vi "LJM_AddressesToMBFB.vi"(1 "NumFrames In (Auto-Detect)":i32=-1, 2 "MaxBytesPerPacket":i32, 5 "aAddresses":i32[](array[numeric]), 7 "aTypes":i32[](array[numeric]), 9 "aValuesIn":dbl[](array[numeric]) format="%.2f", 11 "error in":errorcluster, 12 "aWrites":i32[](array[ring]) items=["Read", "Write"], 13 "aNumValues":i32[](array[numeric])) -> (3 "NumFrames Out":i32, 10 "MBFBCommand":u8[](array[numeric]), 15 "error out":errorcluster)   [LabVIEW 2020]
uses:
  LabJackM.framework
panel:
  # "1/20/2015:  Default value of NumFrames changed to -1 which\nequates to Auto-Detect.  If NumFrames = -1, then the NumFrames\ncontrol is ignored and the size of aNames/aAddresses is used to\ndetermine how many frames there are."
  # "0 => 62"
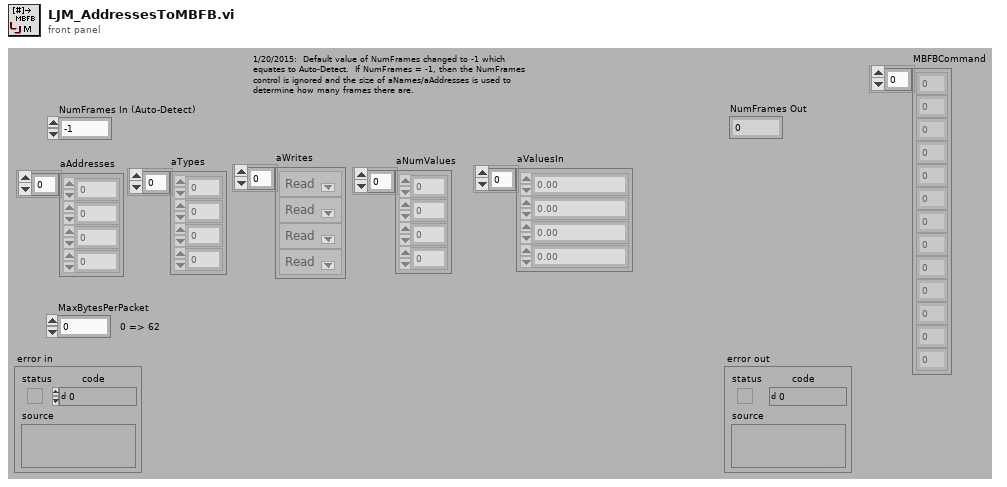
[diagram p1: front panel]
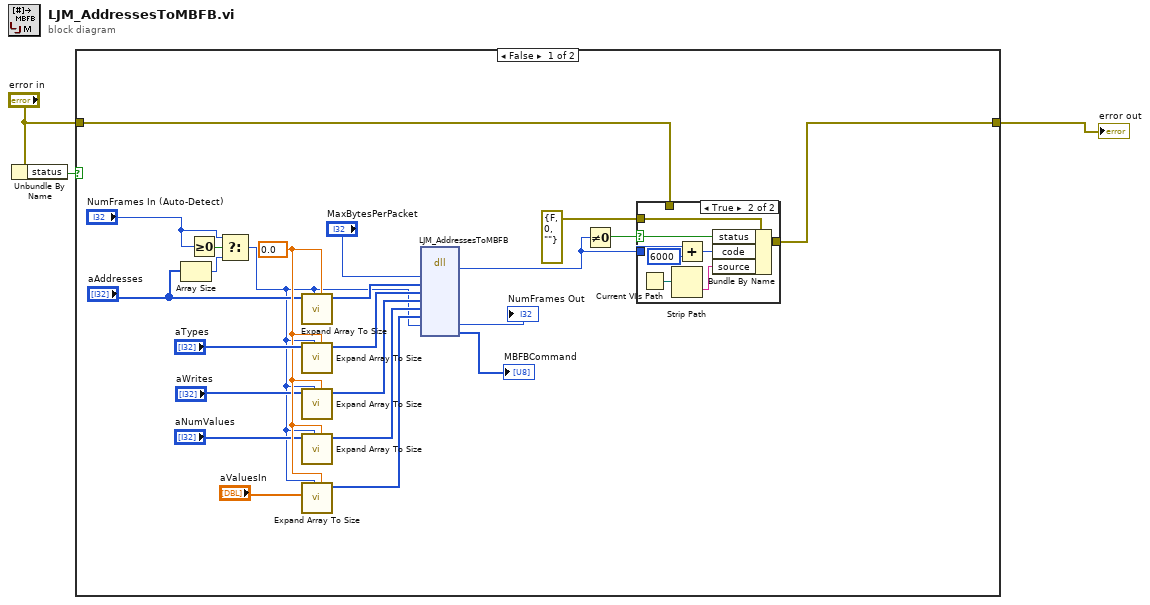
[diagram p0: block diagram]
diagram:
  n1 = Unbundle By Name("error in") -> ("status"=w3:bool)
  n2 = case shown="False" w3 {
    tunnel: "error in" -> [w23 w36]
    tunnel: [w22 w36] -> w1
    frame False {
      w19 = 0.0 ("Default Value")
      n3 = Array Size(array="aAddresses") -> (size(s)=w8:i32)
      n4 = Greater Or Equal To 0?(x="NumFrames In (Auto-Detect)") -> (x >= 0?=w7:bool)
      n5 = Select(t="NumFrames In (Auto-Detect)", s=w7, f=w8) -> (s? t:f=w4:i32)
      n6 = call "Expand Array To Size.vi"("Default Value"=w19, "# Elements"=w4, "I32 Array In"="aAddresses") -> ("I32 Array Out"=w16:i32[])  [unwired: 4 in, 4 out]
      n7 = call "Expand Array To Size.vi"("Default Value"=w19, "# Elements"=w4, "I32 Array In"="aTypes") -> ("I32 Array Out"=w15:i32[])  [unwired: 4 in, 4 out]
      n8 = call "Expand Array To Size.vi"("Default Value"=w19, "# Elements"=w4, "I32 Array In"="aWrites") -> ("I32 Array Out"=w14:i32[])  [unwired: 4 in, 4 out]
      n9 = call "Expand Array To Size.vi"("Default Value"=w19, "# Elements"=w4, "I32 Array In"="aNumValues") -> ("I32 Array Out"=w13:i32[])  [unwired: 4 in, 4 out]
      n10 = call "Expand Array To Size.vi"("Default Value"=w19, "# Elements"=w4, "DBL Array In"="aValuesIn") -> ("I32 Array Out"=w12:i32[])  [unwired: 4 in, 4 out]
      n11 = dll-call lib="LabJackM.framework" fn="LJM_AddressesToMBFB"("MaxBytesPerMBFB"="MaxBytesPerPacket", "aAddresses"=w16, "aTypes"=w15, "aWrites"=w14, "aNumValues"=w13, "aValues"=w12, "NumFrames"=w4) -> ("return type"=w26:i32, "NumFrames"=→"NumFrames Out":i32, "aMBFBCommand"=→"MBFBCommand":u8[])  [unwired: 10 in, 2 out]
      n12 = Not Equal To 0?(x=w26) -> (x != 0?=w25:bool)
      n13 = case shown="True" w25 {
        selector: w25 -> [_ w34]
        tunnel: [w27 w35] -> w22
        tunnel: errorcluster {"status"=FALSE, "code"=0, "source"=""} ("error IO") -> [_ w33]
        tunnel: w26 -> [_ w29]
        tunnel: w23 -> [w27 _]
        frame False {
        }
        frame True {
          n14 = Current VI's Path() -> (path=w31:path)
          n15 = Strip Path(path=w31) -> (name=w32:string)  [unwired: 1 out]
          n16 = Add(x=w29, y=6000) -> (x+y=w30:i32)
          n17 = Bundle By Name(cluster=w33, "status"=w34, "code"=w30, "source"=w32) -> (w35:errorcluster)
        }
      }
    }
    frame True {
    }
  }
  "error out" <- w1
